vi "Caller.vi"(0 "VI Path":path, 5 "Call":bool, 7 "Abort":bool, 9 "error in (no error)":errorcluster) -> (4 "error out":errorcluster)   [LabVIEW 2020]
doc: "This VI calls the selected VI when the CALL button is pressed and aborts this VI whenever the ABORT button is pressed."
panel:
  # "1)Select .vi file in the VI Path.\n2)Press \"CALL\" to open the selected VI and run it.\n3)Press \"ABORT\" to abort the \"Caller\" VI"
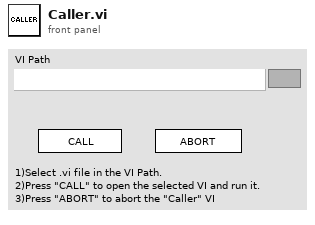
[diagram p1: front panel]
types:
  T1 = enum32{"Invalid", "Standard", "Closed", "Hidden", "Minimized", "Maximized"}
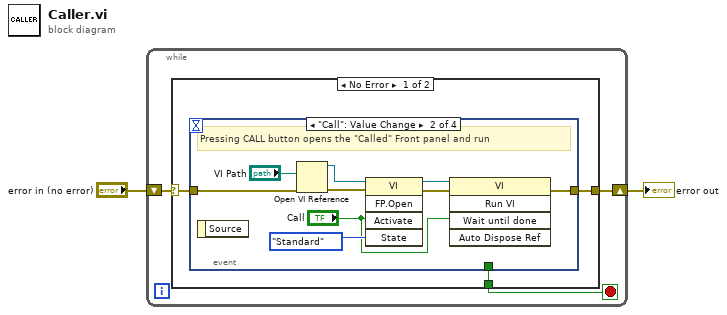
[diagram p0: block diagram]
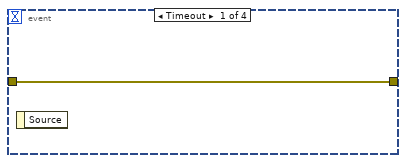
[diagram p2: hidden frame]
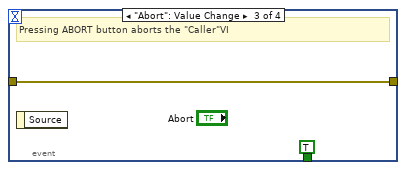
[diagram p3: hidden frame]
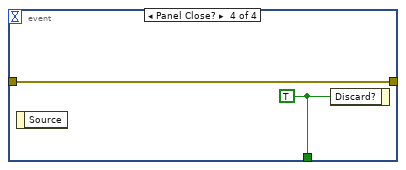
[diagram p4: hidden frame]
diagram:
  n1 = while {
    shift-right: [w5] -> w2
    shift-left: "error in (no error)" -> [w4]
    stop <- w3 stop-if-true
    n2 = case shown="No Error" w4 {
      selector: w4 -> [w6 w23]
      tunnel: [w8 w23] -> w5
      tunnel: [w7 _] -> w3
      frame No Error {
        n3 = event shown="[1] \"Call\": Value Change" {
          selector: _ -> [_ _ _ _]
          dyn-events: _ -> [_ _ _ _]
          timeout: _ -> [_ _ _ _]
          tunnel: [w9 w16 w19 w21] -> w8
          tunnel: [_ _ TRUE ("Discard?") w22] -> w7
          tunnel: w6 -> [w9 w12 w19 w21]
          event Timeout {
            n4 = event-data() -> ()  [unwired: 1 in, 1 out]
          }
          event "Call": Value Change {
            # "Pressing CALL button opens the \"Called\" Front panel and run"
            n5 = event-data() -> ()  [unwired: 1 in, 1 out]
            n6 = Open VI Reference(vi path="VI Path", error in (no error)=w12) -> (vi reference=w13:refnum<vi>, error out=w14:errorcluster)  [unwired: 4 in]
            n7 = invoke class="VI" method="FP.Open"(reference=w13, error in=w14, "Activate"="Call", "State"=T1."Standard") -> (reference out=w18:refnum<vi>, error out=w17:errorcluster)  [unwired: 1 in, 3 out]
            n8 = invoke class="VI" method="Run VI"(reference=w18, error in=w17, "Wait until done"="Call") -> (error out=w16:errorcluster)  [unwired: 2 in, 4 out]
          }
          event "Abort": Value Change {
            # "Pressing ABORT button aborts the \"Caller\"VI"
            n9 = event-data() -> ()  [unwired: 1 in, 1 out]
          }
          event Panel Close? {
            w22 = TRUE ("Discard?")
            n10 = event-data() -> ()  [unwired: 1 in, 1 out]
            n11 = event-data("Discard?"=w22) -> ()  [unwired: 1 in, 1 out]
          }
        }
      }
      frame Error {
      }
    }
  }
  "error out" <- w2
